vi "Run Step.vi"(0 "CAN Cmd Ref":refnum<vi>, 2 "FPGA Ref":T2, 3 "Stagger Time (ms)":i32, 4 "Cycles Completed in":u32, 5 "PWM Freq (Hz)":dbl, 7 "Controller Type:":T3, 8 "# of Steps":i32, 9 "Restarts Cluster":T4={"CMD Starts:"=[0, 0, 0, 0, 0, 0], "Restarts:"=[0, 0, 0, 0, 0, 0], "Total CMD:"=[0, 0, 0, 0, 0, 0], "Total Restarts:"=[0, 0, 0, 0, 0, 0]}, 10 "VoltCtrlRef":string, 13 "Stagger Counter":i32, 14 "Current Step in":i32, 15 "Last CMDs":dbl[](array[numeric]), 16 "Profile":string[][](array[string]), 17 "Pumps Present":u32) -> (12 "PS Cmd":dbl, 19 "Ignition Relays":T1, 20 "Manual CMDs":dbl[](array[numeric]), 21 "Current Step out":i32, 23 "Press Cmd":dbl, 24 "Cycles Completed out":u32, 25 "Step Time":dbl, 26 "Power Relays":T1, 27 "Restarts Cluster OUT":T4)   [LabVIEW 2013]
uses:
  Type Defs/Restarts Cluster.ctl
  Type Defs/Controller Names.ctl
  Controls/FPGA_Reference.ctl
  <vilib>/Utility/error.llb/Error Cluster From Error Code.vi
  <vilib>/rvi/errors/niLvFpgaAdjustHostInterfaceError.vi
  <vilib>/rvi/interface/nirviReadWriteControl/nirviReadWriteControl.xnode
  FPGA/bitfiles/TI sbRIO PWM (FPGA) v1.0.lvbitx
  FPGA/TI sbRIO Main (FPGA).vi
  NiFpgaLv.dll
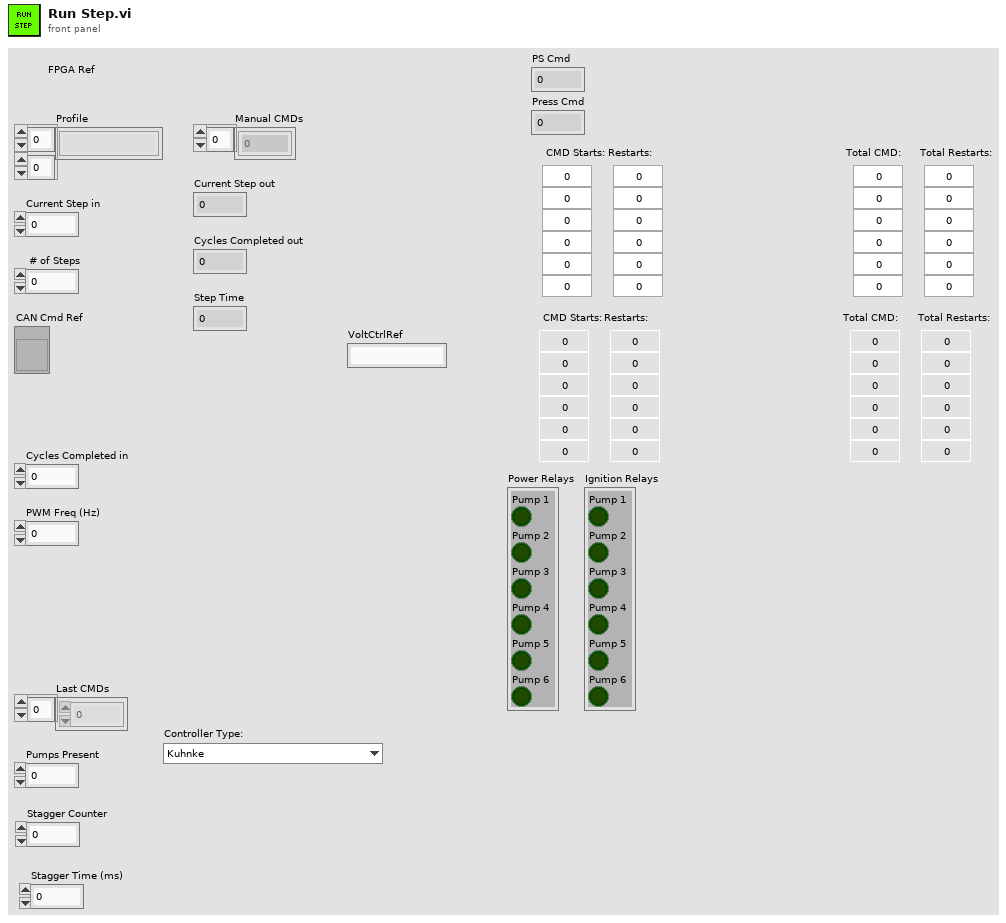
[diagram p1: front panel]
types:
  T1 = cluster{"Pump 1":bool, "Pump 2":bool, "Pump 3":bool, "Pump 4":bool, "Pump 5":bool, "Pump 6":bool}
  T2 = typedef "FPGA_Reference.ctl" = refnum<k20>
  T3 = typedef "Controller Names.ctl" = enum16{"Kuhnke", "Conti", "Helbako", "TI PWM", "PSA", "Hella Gas", "Hella Diesel", "8 Comm", "10 Comm", "8 Comm Hella", "10 Comm Hella", "8 Comm Omron", "10 Comm Omron", "8 Comm Nissan", "10 Comm Nissan"}
  T4 = typedef "Restarts Cluster.ctl" = cluster{"CMD Starts:":i32[], "Restarts:":i32[], "Total CMD:":i32[], "Total Restarts:":i32[]}
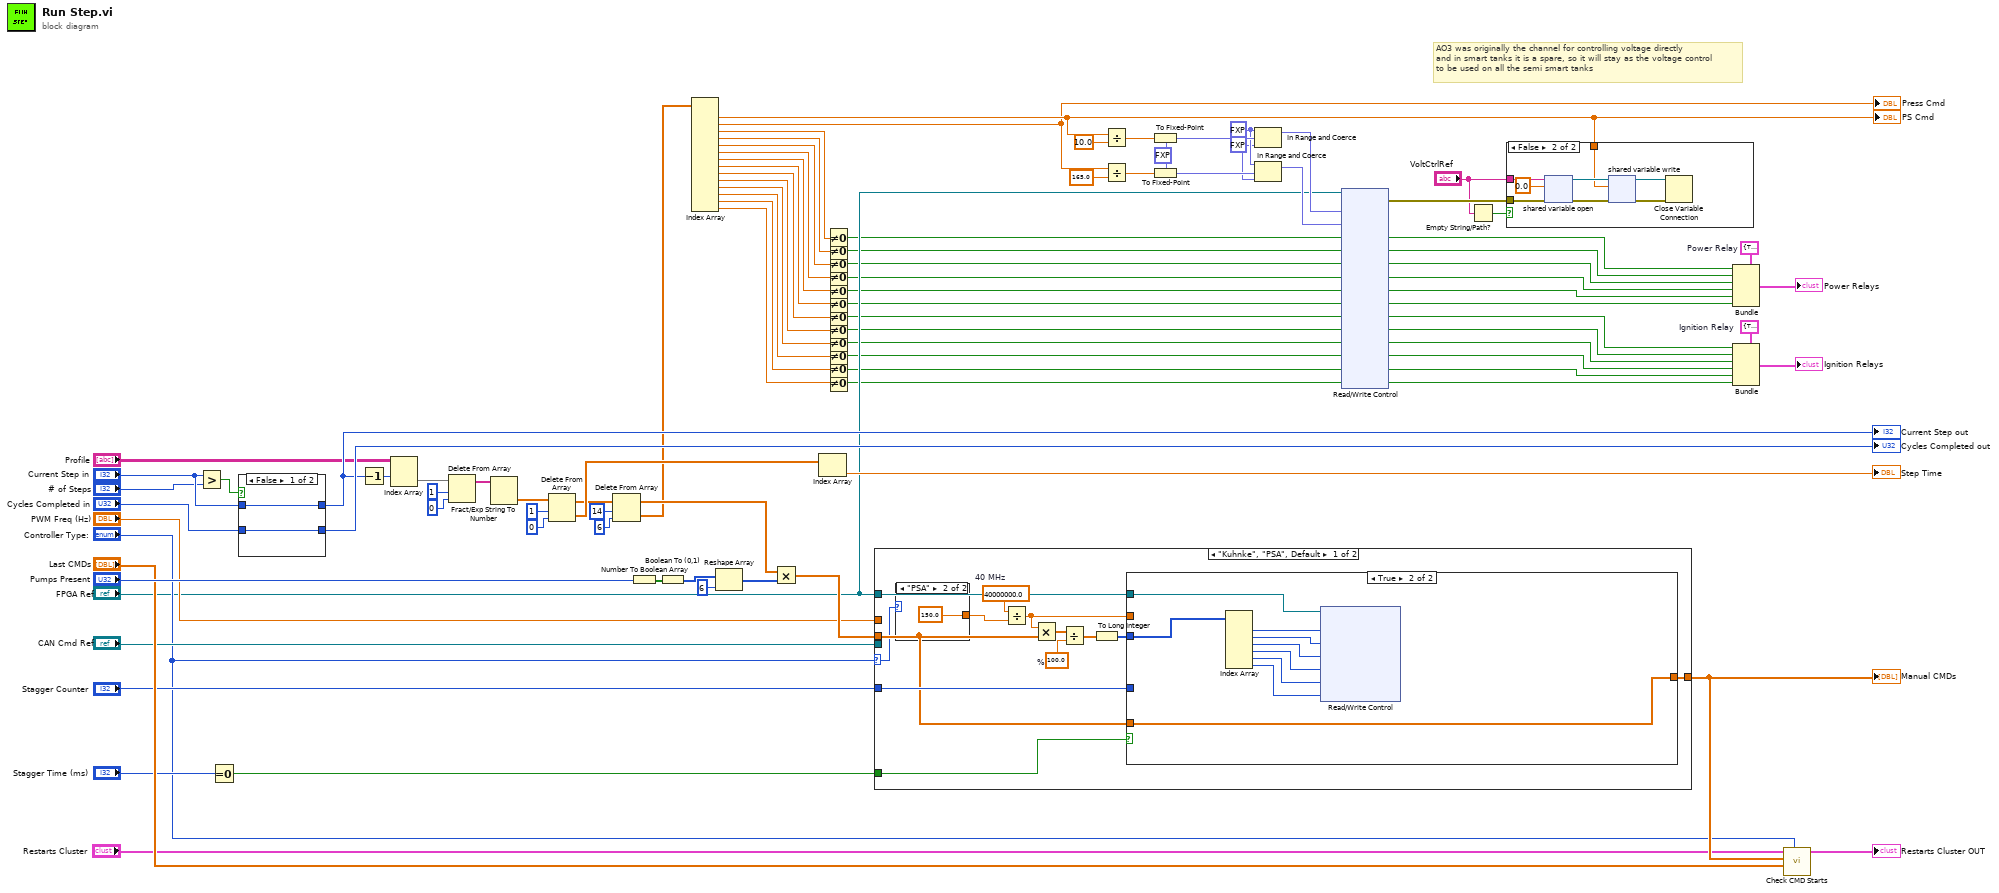
[diagram p0: block diagram]
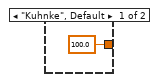
[diagram p3: hidden frame]
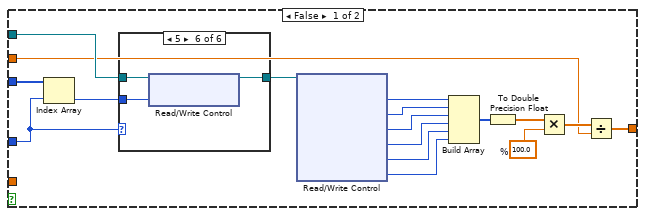
[diagram p4: hidden frame]
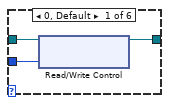
[diagram p5: hidden frame]
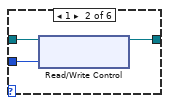
[diagram p6: hidden frame]
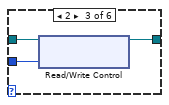
[diagram p7: hidden frame]
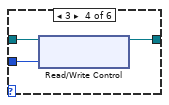
[diagram p8: hidden frame]
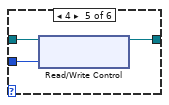
[diagram p9: hidden frame]
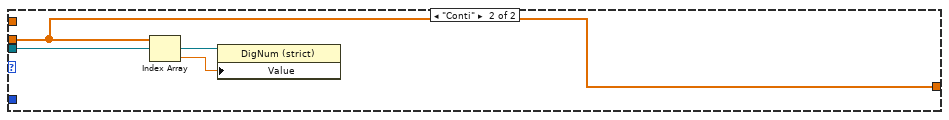
[diagram p10: hidden frame]
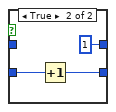
[diagram p11: hidden frame]
diagram:
  w18 = T1 {"Pump 1"=TRUE, "Pump 2"=TRUE, "Pump 3"=TRUE, "Pump 4"=TRUE, "Pump 5"=TRUE, "Pump 6"=TRUE}  # Ignition Relay
  w19 = T1 {"Pump 1"=TRUE, "Pump 2"=TRUE, "Pump 3"=TRUE, "Pump 4"=TRUE, "Pump 5"=TRUE, "Pump 6"=TRUE}  # Power Relay
  w38 = fxp<+/-,20,5> 0.0 ("lower limit")
  w39 = fxp<+/-,20,5> 5.0 ("upper limit")
  w51 = fxp<+/-,20,5> 0.0 ("AO0")
  # "AO3 was originally the channel for controlling voltage directly\nand in smart tanks it is a spare, so it will stay as the voltage control\nto be used on all the semi smart tanks"
  n1 = Greater?(x="Current Step in", y="# of Steps") -> (0:w76:bool)
  n2 = Equal To 0?(x="Stagger Time (ms)") -> (x = 0?=w54:bool)
  n3 = case shown="False" w76 {
    tunnel: [w85 1 ("Current Step")] -> w78
    tunnel: "Current Step in" -> [w85 _]
    tunnel: "Cycles Completed in" -> [w84 w87]
    tunnel: [w84 w86] -> w80
    frame False {
    }
    frame True {
      n4 = Increment(x=w87) -> (x+1=w86:u32)
    }
  }
  "Cycles Completed out" <- w80
  "Current Step out" <- w78
  n5 = Decrement(x=w78) -> (x-1=w64:i32)
  n6 = Index Array(array="Profile", index (row)=w64) -> (element=w65:string[])  [unwired: 1 in]
  n7 = Delete From Array(array=w65, length=1, index=0 ("length")) -> (array with subset deleted=w69:string[])  [unwired: 1 out]
  n8 = Fract/Exp String To Number(string=w69) -> (number=w72:dbl[])  [unwired: 3 in, 1 out]
  n9 = Delete From Array(array=w72, length=1, index=0 ("length")) -> (deleted portion=w73:dbl[], array with subset deleted=w61:dbl[])
  n10 = Delete From Array(array=w61, length=14, index=6) -> (deleted portion=w49:dbl[], array with subset deleted=w58:dbl[])
  n11 = Number To Boolean Array(number="Pumps Present") -> (Boolean array=w50:bool[])
  n12 = Boolean To (0,1)(Boolean=w50) -> (0, 1=w3:i16[])
  n13 = Index Array(array=w49) -> (element #1=w32:dbl, element #2=w31:dbl, element #3=w48:dbl, element #4=w30:dbl, element #5=w28:dbl, element #6=w29:dbl, element #7=w27:dbl, element #8=w26:dbl, element #9=w25:dbl, element #10=w23:dbl, element #11=w24:dbl, element #12=w22:dbl, element #13=w21:dbl, element #14=w20:dbl)  [unwired: 14 in]
  "PS Cmd" <- w32
  "Press Cmd" <- w31
  n14 = Reshape Array(w3, 6 ("dimension size")) -> (w2:i16[])
  n15 = Multiply(x=w58, y=w2) -> (x*y=w83:dbl[])
  n16 = Index Array(array=w73) -> (element=→"Step Time":dbl)  [unwired: 1 in]
  n17 = Not Equal To 0?(x=w48) -> (x != 0?=w17:bool)
  n18 = Not Equal To 0?(x=w30) -> (x != 0?=w16:bool)
  n19 = Not Equal To 0?(x=w28) -> (x != 0?=w15:bool)
  n20 = Not Equal To 0?(x=w29) -> (x != 0?=w14:bool)
  n21 = Not Equal To 0?(x=w27) -> (x != 0?=w13:bool)
  n22 = Not Equal To 0?(x=w26) -> (x != 0?=w12:bool)
  n23 = Not Equal To 0?(x=w25) -> (x != 0?=w11:bool)
  n24 = Not Equal To 0?(x=w23) -> (x != 0?=w10:bool)
  n25 = Not Equal To 0?(x=w24) -> (x != 0?=w9:bool)
  n26 = Not Equal To 0?(x=w22) -> (x != 0?=w7:bool)
  n27 = Not Equal To 0?(x=w21) -> (x != 0?=w8:bool)
  n28 = Not Equal To 0?(x=w20) -> (x != 0?=w6:bool)
  n29 = case shown="\"Kuhnke\", \"PSA\", Default" "Controller Type:" {
    selector: "Controller Type:" -> [w90 _]
    tunnel: "PWM Freq (Hz)" -> [_ _]
    tunnel: w83 -> [w91 w148]
    tunnel: "FPGA Ref" -> [w96 _]
    tunnel: "CAN Cmd Ref" -> [_ w149]
    tunnel: "Stagger Counter" -> [w95 _]
    tunnel: [w93 w148] -> w56
    tunnel: w54 -> [w92 _]
    frame "Kuhnke", "PSA", Default {
      w100 = 40000000.0  # 40 MHz
      w98 = 100.0  # %
      n30 = case shown="\"PSA\"" w90 {
        tunnel: [100.0 ("y") 150.0 ("y")] -> w89
        frame "Kuhnke", Default {
        }
        frame "PSA" {
        }
      }
      n31 = Divide(x=w100, y=w89) -> (x/y=w94:dbl)
      n32 = Multiply(x=w94, y=w91) -> (x*y=w97:dbl[])
      n33 = Divide(x=w97, y=w98) -> (x/y=w99:dbl[])
      n34 = To Long Integer(number=w99) -> (32bit integer=w101:i32[])
      n35 = case shown="True" w92 {
        tunnel: w101 -> [w120 w147]
        tunnel: w96 -> [w119 w139]
        tunnel: w95 -> [w117 _]
        tunnel: w94 -> [w105 _]
        tunnel: [w104 w146] -> w93
        tunnel: w91 -> [_ w146]
        frame False {
          w107 = 100.0  # %
          n36 = Index Array(array=w120, index=w117) -> (element=w118:i32)
          n37 = case shown="5" w117 {
            tunnel: w119 -> [w123 w126 w129 w132 w135 w138]
            tunnel: w118 -> [w122 w125 w128 w131 w134 w137]
            tunnel: [w121 w124 w127 w130 w133 w136] -> w116
            frame 0, Default {
              n38 = xnode "Read/Write Control"("FPGA VI Reference In"=w123, "Duty (Ticks) 1"=w122) -> ("FPGA VI Reference Out"=w121:T2)  [unwired: 1 in, 1 out]
            }
            frame 1 {
              n39 = xnode "Read/Write Control"("FPGA VI Reference In"=w126, "Duty (Ticks) 2"=w125) -> ("FPGA VI Reference Out"=w124:T2)  [unwired: 1 in, 1 out]
            }
            frame 2 {
              n40 = xnode "Read/Write Control"("FPGA VI Reference In"=w129, "Duty (Ticks) 3"=w128) -> ("FPGA VI Reference Out"=w127:T2)  [unwired: 1 in, 1 out]
            }
            frame 3 {
              n41 = xnode "Read/Write Control"("FPGA VI Reference In"=w132, "Duty (Ticks) 4"=w131) -> ("FPGA VI Reference Out"=w130:T2)  [unwired: 1 in, 1 out]
            }
            frame 4 {
              n42 = xnode "Read/Write Control"("FPGA VI Reference In"=w135, "Duty (Ticks) 5"=w134) -> ("FPGA VI Reference Out"=w133:T2)  [unwired: 1 in, 1 out]
            }
            frame 5 {
              n43 = xnode "Read/Write Control"("FPGA VI Reference In"=w138, "Duty (Ticks) 6"=w137) -> ("FPGA VI Reference Out"=w136:T2)  [unwired: 1 in, 1 out]
            }
          }
          n44 = xnode "Read/Write Control"("FPGA VI Reference In"=w116) -> ("Duty (Ticks) 1"=w115:i32, "Duty (Ticks) 2"=w114:i32, "Duty (Ticks) 3"=w113:i32, "Duty (Ticks) 4"=w112:i32, "Duty (Ticks) 5"=w111:i32, "Duty (Ticks) 6"=w110:i32)  [unwired: 1 in, 2 out]
          n45 = Build Array(w115, w114, w113, w112, w111, w110) -> (w109:i32[])
          n46 = To Double Precision Float(number=w109) -> (double precision float=w108:dbl[])
          n47 = Multiply(x=w108, y=w107) -> (x*y=w106:dbl[])
          n48 = Divide(x=w106, y=w105) -> (x/y=w104:dbl[])
        }
        frame True {
          n49 = Index Array(array=w147) -> (element #1=w145:i32, element #2=w144:i32, element #3=w143:i32, element #4=w142:i32, element #5=w141:i32, element #6=w140:i32)  [unwired: 6 in]
          n50 = xnode "Read/Write Control"("FPGA VI Reference In"=w139, "Duty (Ticks) 1"=w145, "Duty (Ticks) 2"=w144, "Duty (Ticks) 3"=w143, "Duty (Ticks) 4"=w142, "Duty (Ticks) 5"=w141, "Duty (Ticks) 6"=w140) -> ()  [unwired: 1 in, 2 out]
        }
      }
    }
    frame "Conti" {
      n51 = Index Array(array=w148) -> (element=w150:dbl)  [unwired: 1 in]
      n52 = property class="DigNum (strict)"(reference=w149, "Value"=w150) -> ()  [unwired: 1 in, 2 out]
    }
  }
  "Manual CMDs" <- w56
  n53 = Divide(x=w32, y=10.0) -> (x/y=w42:dbl)
  n54 = Divide(x=w31, y=165.0) -> (x/y=w43:dbl)
  n55 = To Fixed-Point(fixed-point type=w51, number=w42) -> (fixed-point=w47:fxp<+/-,20,5>)
  n56 = To Fixed-Point(fixed-point type=w51, number=w43) -> (fixed-point=w46:fxp<+/-,20,5>)
  n57 = In Range and Coerce(upper limit=w39, x=w47, lower limit=w38) -> (coerced(x)=w40:fxp<+/-,20,5>)  [unwired: 1 out]
  n58 = In Range and Coerce(upper limit=w39, x=w46, lower limit=w38) -> (coerced(x)=w41:fxp<+/-,20,5>)  [unwired: 1 out]
  n59 = xnode "Read/Write Control"("FPGA VI Reference In"="FPGA Ref", "AO3"=w40, "AO0"=w41, "DIO6"=w17, "DIO7"=w16, "DIO8"=w15, "DIO9"=w14, "DIO10"=w13, "DIO11"=w12, "DIO12"=w11, "DIO13"=w10, "DIO14"=w9, "DIO15"=w7, "DIO16"=w8, "DIO17"=w6) -> ("error out"=w36:errorcluster)  [unwired: 1 in, 1 out]
  n60 = Empty String/Path?(string/path="VoltCtrlRef") -> (empty?=w37:bool)
  n61 = case shown="False" w37 {
    tunnel: w36 -> [_ w154]
    tunnel: w32 -> [_ w152]
    tunnel: "VoltCtrlRef" -> [_ w151]
    frame True {
    }
    frame False {
      n62 = shared-variable-open(w151, w154, 0.0) -> (w158:refnum<k21>, w155:errorcluster)  [unwired: 1 in]
      n63 = shared-variable-write(w158, w155, w152) -> (w157:refnum<k21>, w156:errorcluster)
      n64 = Close Variable Connection(8:w156, 11:w157) -> ()  [unwired: 1 out]
    }
  }
  n65 = Bundle(cluster=w19, "Pump 1"=w17, "Pump 2"=w16, "Pump 3"=w15, "Pump 4"=w14, "Pump 5"=w13, "Pump 6"=w12) -> (→"Power Relays":T1)
  n66 = Bundle(cluster=w18, "Pump 1"=w11, "Pump 2"=w10, "Pump 3"=w9, "Pump 4"=w7, "Pump 5"=w8, "Pump 6"=w6) -> (→"Ignition Relays":T1)
  n67 = call "Check CMD Starts.vi"("Controller Type:"="Controller Type:", "Last CMDs"="Last CMDs", "Current CMDs"=w56, "Restarts Cluster IN"="Restarts Cluster") -> ("Restarts Cluster OUT"=→"Restarts Cluster OUT":T4)  [unwired: 7 in]
